vi "2023 FMS Arm and Wrist Controller.vi"(3 "error in":errorcluster, 4 "armMotorControlDevRef":T1, 5 "wristMotorControlDevRef":T1) -> (0 "error out":errorcluster, 1 "armSensorPosition":dbl, 2 "wristSensorPosition":dbl)   [LabVIEW 2020]
uses:
  <vilib>/Rock Robotics/WPI/MotorControl/WPI_MotorControlDeviceRef.ctl
  <vilib>/Rock Robotics/WPI/MotorControl/WPI_MotorControlType.ctl
  <vilib>/Rock Robotics/SystemInterfaces/DIO/FPGA_DIOPWMChannel.ctl
  <vilib>/Rock Robotics/WPI/PWM/WPI_PWMDeadband.ctl
  <vilib>/Rock Robotics/SystemInterfaces/DIO/FPGA_DIOChannel.ctl
  2023 Robot Global Data.vi
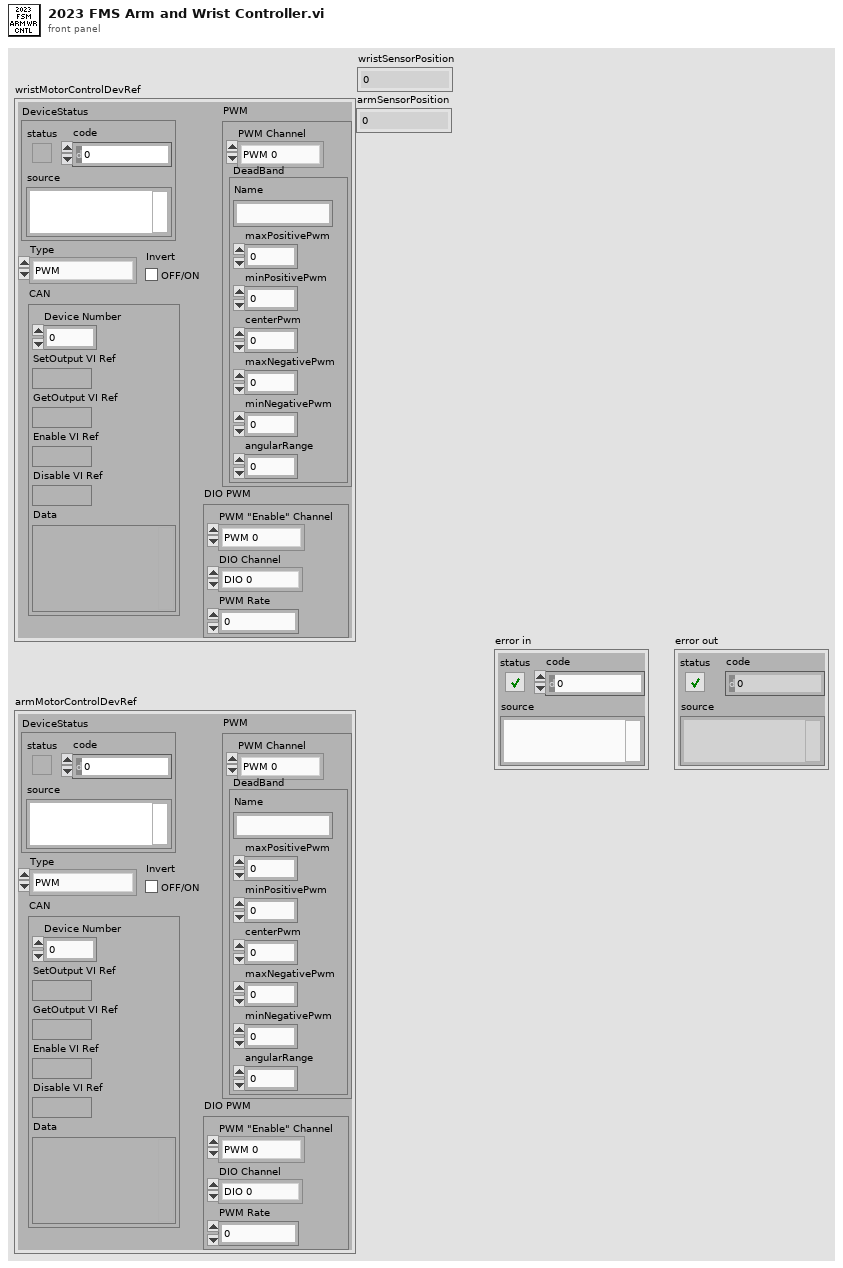
[diagram p1: front panel]
types:
  T1 = typedef "WPI_MotorControlDeviceRef.ctl" = cluster{"DeviceStatus":errorcluster, "Type":T2, "PWM":cluster{"PWM Channel":T3, "DeadBand":T4}, "CAN":cluster{"Device Number":u8, "SetOutput VI Ref":variant, "GetOutput VI Ref":variant, "Enable VI Ref":variant, "Disable VI Ref":variant, "Data":variant}, "Invert":bool, "DIO PWM":cluster{"PWM \"Enable\" Channel":T3, "DIOChannel":T5, "PWM Rate":dbl}}
  T2 = typedef "WPI_MotorControlType.ctl" = enum16{"PWM", "CAN", "DIO PWM"}
  T3 = typedef "FPGA_DIOPWMChannel.ctl" = enum8{"PWM 0", "PWM 1", "PWM 2", "PWM 3", "PWM 4", "PWM 5", "PWM 6", "PWM 7", "PWM 8", "PWM 9", "PWM MXP 0", "PWM MXP 1", "PWM MXP 2", "PWM MXP 3", "PWM MXP 4", "PWM MXP 5", "PWM MXP 6", "PWM MXP 7", "PWM MXP 8", "PWM MXP 9", "Invalid"}
  T4 = typedef "WPI_PWMDeadband.ctl" = cluster{"Name":string, "maxPositivePwm":i32, "minPositivePwm":i32, "centerPwm":i32, "maxNegativePwm":i32, "minNegativePwm":i32, "angularRange":u16}
  T5 = typedef "FPGA_DIOChannel.ctl" = enum8{"DIO 0", "DIO 1", "DIO 2", "DIO 3", "DIO 4", "DIO 5", "DIO 6", "DIO 7", "DIO 8", "DIO 9", "DIO MXP 0", "DIO MXP 1", "DIO MXP 2", "DIO MXP 3", "DIO MXP 4", "DIO MXP 5", "DIO MXP 6", "DIO MXP 7", "DIO MXP 8", "DIO MXP 9", "DIO MXP 10", "DIO MXP 11", "DIO MXP 12", "DIO MXP 13", "DIO MXP 14", "DIO MXP 15", "SPI Port CS1", "SPI Port CS2", "SPI Port CS3", "SPI Port MISO", "SPI Port MOSI", "Invalid"}
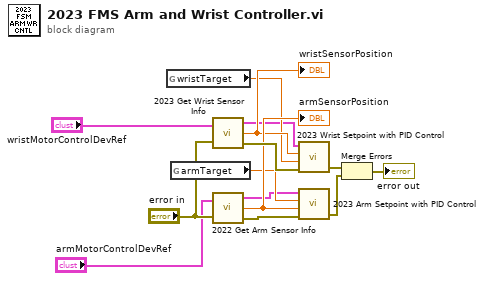
[diagram p0: block diagram]
diagram:
  n1 = global read "2023 Robot Global Data.vi" "wristTarget"() -> (w9:dbl)
  n2 = global read "2023 Robot Global Data.vi" "armTarget"() -> (w10:dbl)
  n3 = call "2023 Get Wrist Sensor Info.vi"("MotorControlDevRefIn"="wristMotorControlDevRef", "error in"="error in") -> ("MotorControlDevRefOut"=w2:T1, "wristSensorPosition"=w11:dbl, "error out"=w14:errorcluster)
  "wristSensorPosition" <- w11
  n4 = call "2022 Get Arm Sensor Info.vi"("MotorControlDevRefIn"="armMotorControlDevRef", "error in (no error)"="error in") -> ("MotorControlDevRefOut"=w1:T1, "armSensorPosition"=w12:dbl, "error out"=w6:errorcluster)
  "armSensorPosition" <- w12
  n5 = call "2023 Wrist Setpoint with PID Control.vi"("error in (no error)"=w14, "wristSetPoint"=w9, "wristSensorPosition"=w11, "MotorControlDevRef"=w2) -> ("error out"=w5:errorcluster)  [unwired: 2 out]
  n6 = call "2023 Arm Setpoint with PID Control.vi"("error in (no error)"=w6, "armSensorPosition"=w12, "armSetpoint"=w10, "MotorControlDevRef"=w1) -> ("error out"=w4:errorcluster)  [unwired: 2 out]
  n7 = Merge Errors(w5, w4) -> (→"error out":errorcluster)
